vi "Compute Convex Hull from points.vi"(1 "Convex Hull Interior":T1[][](array[typedef])) -> (0 "Convex Hull Regions":T1[](array[typedef]))   [LabVIEW 2018]
uses:
  Classes/Video Cam Processor/Private/Hull Point STYP.ctl
  <vilib>/Analysis/NI_AAL_Geometry.lvlib
  Classes/Video Cam Processor/Video Cam Processor.lvclass
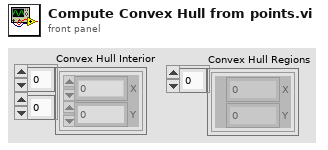
[diagram p1: front panel]
types:
  T1 = typedef "Video Cam Processor.lvclass/Hull Point STYP.ctl" = cluster{"X":i32, "Y":i32}
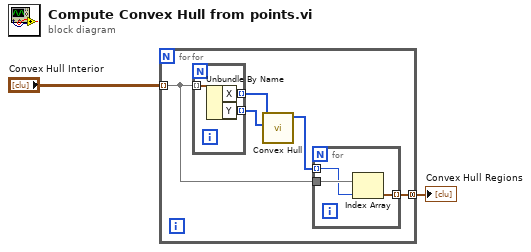
[diagram p0: block diagram]
diagram:
  n1 = for {
    tunnel: "Convex Hull Interior" -> [w4] mode=indexing
    tunnel: [w3] -> w1 mode=concatenating
    n2 = for {
      tunnel: w4 -> [w13] mode=indexing
      tunnel: [w12] -> w7 mode=indexing
      tunnel: [w11] -> w6 mode=indexing
      n3 = Unbundle By Name(w13) -> ("X"=w12:i32, "Y"=w11:i32)
    }
    n4 = call <vilib>:"Convex Hull.vi"("Y"=w6, "X"=w7) -> ("Convex Hull"=w5:i32[])  [unwired: 8 in, 1 out]
    n5 = for {
      tunnel: w5 -> [w9] mode=indexing
      tunnel: w4 -> [w10]
      tunnel: [w8] -> w3 mode=indexing
      n6 = Index Array(array=w10, index=w9) -> (element=w8:T1)
    }
  }
  "Convex Hull Regions" <- w1
